vi "get_active_channels.vi"(7 "Trigger edge":bool[](array[boolean])=[FALSE, FALSE, FALSE, FALSE, FALSE, FALSE, FALSE, FALSE], 8 "Error In":errorcluster, 9 "swabian_local_data":T1={"events"={"update_status"=refnum, "update_chart"=refnum, "update_xy"=refnum, "send_channel_data"=refnum}, "stop_q"=refnum, "tagger_reference"=refnum, "connect_button"=refnum, "counter_reference"=refnum, "tagger_stream_reference"=refnum, "log_reference"=refnum, "current_log_offset"=0, "tt20_buffer_q"=refnum, "stream_to_file_button"=refnum, "num_records"=0, "connected?"=FALSE, "plots"=refnum, "histogram_bin_edges"=[], "histogrammer"=refnum, "plot_lifetimes"=refnum, "xy_graph"=refnum, "Reference\nChannel"=enum."ch0", "trigger_channels"=[], "filter_channels"=[], "active_channels"=[], "acq_mode"=0, "Reference\nChannel"=enum."ch0", "acq_time"=0, "sync_period_ps"=0, "raw_stream_path"=path "", "Leftovers"={"missing_sync_data"=[], "missing_events"=0}, "first_batch"=0, "first_sync_stamp"=0, "lifetime_settings"={"Plot Lifetimes"=FALSE, "start_time"=0.0, "stop_time"=0.0, "n_bins"=0, "Oscilloscope"=TRUE}, "Histogram_bins"=[], "last_processed_data"=[], "histogram_data"=[]}, 10 "Reference\nChannel":T3=enum."ch2", 11 "channels_to_stream":bool[](array[boolean])) -> (0 "Error In 2":errorcluster, 3 "swabian_local_data 2":T1={"events"={"update_status"=refnum, "update_chart"=refnum, "update_xy"=refnum, "send_channel_data"=refnum}, "stop_q"=refnum, "tagger_reference"=refnum, "connect_button"=refnum, "counter_reference"=refnum, "tagger_stream_reference"=refnum, "log_reference"=refnum, "current_log_offset"=0, "tt20_buffer_q"=refnum, "stream_to_file_button"=refnum, "num_records"=0, "connected?"=FALSE, "plots"=refnum, "histogram_bin_edges"=[], "histogrammer"=refnum, "plot_lifetimes"=refnum, "xy_graph"=refnum, "Reference\nChannel"=enum."ch0", "trigger_channels"=[], "filter_channels"=[], "active_channels"=[], "acq_mode"=0, "Reference\nChannel"=enum."ch0", "acq_time"=0, "sync_period_ps"=0, "raw_stream_path"=path "", "Leftovers"={"missing_sync_data"=[], "missing_events"=0}, "first_batch"=0, "first_sync_stamp"=0, "lifetime_settings"={"Plot Lifetimes"=FALSE, "start_time"=0.0, "stop_time"=0.0, "n_bins"=0, "Oscilloscope"=TRUE}, "Histogram_bins"=[], "last_processed_data"=[], "histogram_data"=[]})   [LabVIEW 2018]
uses:
  reference_checkbox_tdef.ctl
  swabian_local_data_tdef.ctl
  swabian_events_tdef.ctl
  update_chart_tdef.ctl
  channel_data_tdef.ctl
  C:/Users/SWIR TCSPC/Documents/swabian_LV/lib/TTCSharp32.dll
  lib/TTCSharp32.dll
  swabian_buffer_tdef.ctl
  lifetime_settings.ctl
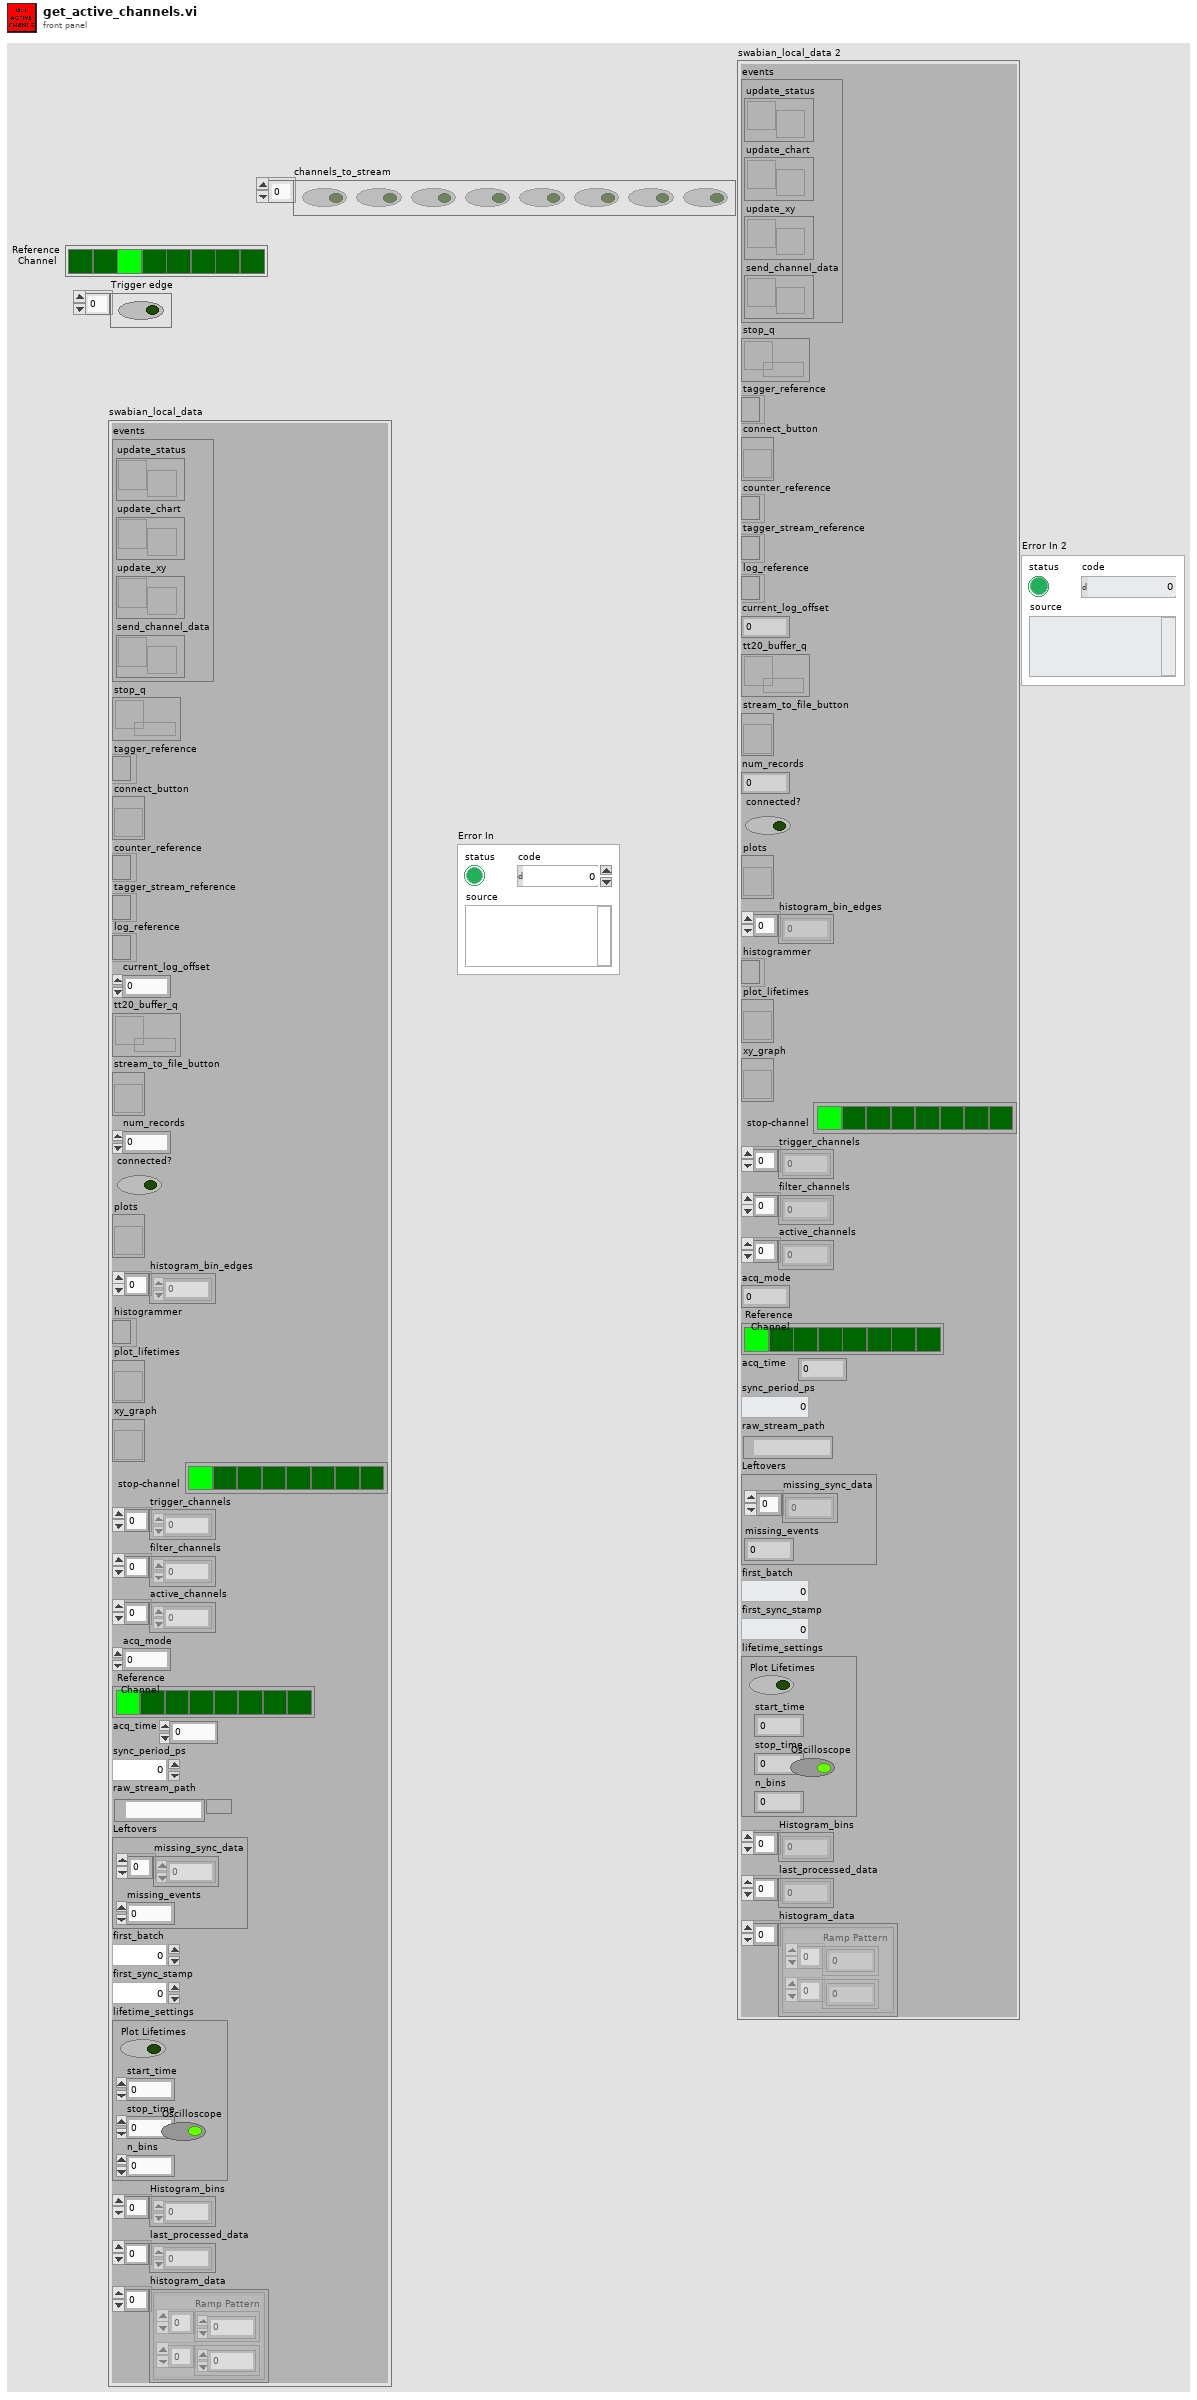
[diagram p1: front panel]
types:
  T1 = typedef "swabian_local_data_tdef.ctl" = cluster{"events":T2, "stop_q":refnum<queue>, "tagger_reference":refnum<k24>, "connect_button":refnum<vi>, "counter_reference":refnum<k24>, "tagger_stream_reference":refnum<k24>, "log_reference":refnum<file>, "current_log_offset":i64, "tt20_buffer_q":refnum<queue>, "stream_to_file_button":refnum<vi>, "num_records":u64, "connected?":bool, "plots":refnum<vi>, "histogram_bin_edges":i64[], "histogrammer":refnum<k24>, "plot_lifetimes":refnum<vi>, "xy_graph":refnum<vi>, "Reference\nChannel":T3, "trigger_channels":i32[], "filter_channels":i32[], "active_channels":i32[], "acq_mode":i32, "Reference\nChannel":T3, "acq_time":i64, "sync_period_ps":i64, "raw_stream_path":path, "Leftovers":cluster{"missing_sync_data":i64[], "missing_events":i32}, "first_batch":i32, "first_sync_stamp":i64, "lifetime_settings":T4, "Histogram_bins":dbl[], "last_processed_data":i64[], "histogram_data":cluster{"Ramp Pattern":dbl[], dbl[]}[]}
  T2 = typedef "swabian_events_tdef.ctl" = cluster{"update_status":refnum<user-event>, "update_chart":refnum<user-event>, "update_xy":refnum<user-event>, "send_channel_data":refnum<user-event>}
  T3 = typedef "reference_checkbox_tdef.ctl" = enum32{"No Selection", "ch0", "ch1", "ch2", "ch3", "ch4", "ch5", "ch6", "ch7"}
  T4 = typedef "lifetime_settings.ctl" = cluster{"Plot Lifetimes":bool, "start_time":dbl, "stop_time":dbl, "n_bins":i32, "Oscilloscope":bool}
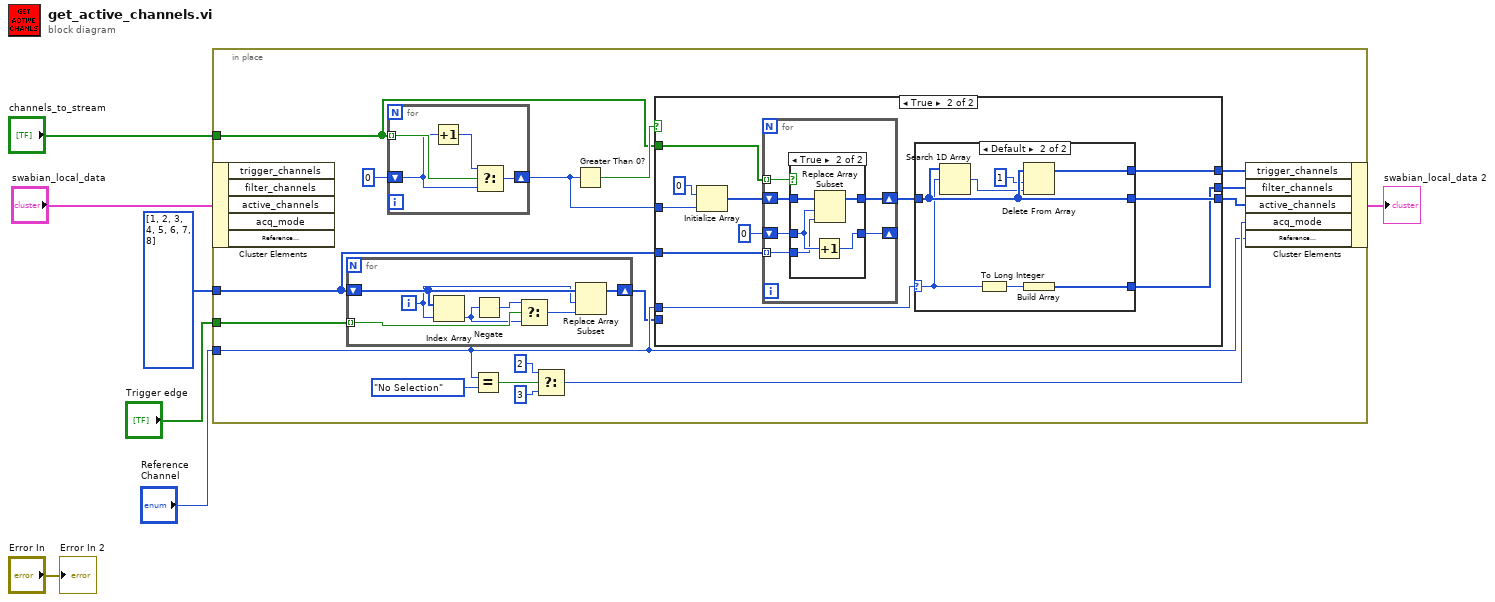
[diagram p0: block diagram]
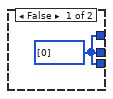
[diagram p2: hidden frame]
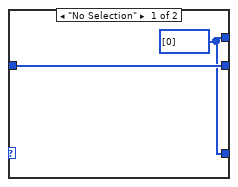
[diagram p4: hidden frame]
diagram:
  n1 = in-place {
    in-place-border: "channels_to_stream" -> [w10]
    in-place-border: "Reference\nChannel" -> [w16]
    in-place-border: i32[] [1, 2, 3, 4, 5, 6, 7, 8] -> [w9]
    in-place-border: "Trigger edge" -> [w15]
    n2 = in-place-cluster #1("swabian_local_data") -> ()  [unwired: 5 out]
    n3 = for {
      tunnel: w15 -> [w68] mode=indexing
      shift-right: [w62] -> w11
      shift-left: w9 -> [w66]
      i -> [w65]
      n4 = Index Array(array=w66, index=w65) -> (element=w64:i32)
      n5 = Negate(x=w64) -> (-x=w63:i32)
      n6 = Select(t=w63, s=w68, f=w64) -> (s? t:f=w67:i32)
      n7 = Replace Array Subset(array=w66, new element=w67, index=w65) -> (w62:i32[])
    }
    n8 = for {
      tunnel: w10 -> [w61] mode=indexing
      shift-right: [w59] -> w12
      shift-left: 0 -> [w58]
      n9 = Increment(x=w58) -> (x+1=w60:i32)
      n10 = Select(t=w60, s=w61, f=w58) -> (s? t:f=w59:i32)
    }
    n11 = Equal?(x=w16, y=reference_checkbox_tdef."No Selection") -> (x = y?=w22:bool)
    n12 = Select(t=2, s=w22, f=3 ("t")) -> (s? t:f=w19:i32)
    n13 = Greater Than 0?(x=w12) -> (x > 0?=w13:bool)
    n14 = case shown="True" w13 {
      tunnel: [w24 w35] -> w8
      tunnel: [w24 w34] -> w18
      tunnel: [w24 w33] -> w17
      tunnel: w16 -> [_ w32]
      tunnel: w12 -> [_ w31]
      tunnel: w11 -> [_ _]
      tunnel: w10 -> [_ w29]
      tunnel: w9 -> [_ w28]
      frame False {
        w24 = i32[] [0]
      }
      frame True {
        n15 = Initialize Array(0 ("element"), w31) -> (w27:i32[])
        n16 = for {
          tunnel: w29 -> [w41] mode=indexing
          tunnel: w28 -> [w39] mode=indexing
          shift-right: [w38] -> w25
          shift-left: w27 -> [w40]
          shift-right: [w36] -> _
          shift-left: 0 -> [w37]
          n17 = case shown="True" w41 {
            tunnel: w40 -> [w43 w48]
            tunnel: w39 -> [_ w44]
            tunnel: [w43 w47] -> w38
            tunnel: w37 -> [w42 w45]
            tunnel: [w42 w46] -> w36
            frame False {
            }
            frame True {
              n18 = Increment(x=w45) -> (x+1=w46:i32)
              n19 = Replace Array Subset(array=w48, new element=w44, index=w45) -> (w47:i32[])
            }
          }
        }
        n20 = case shown="Default" w32 {
          selector: w32 -> [_ w51]
          tunnel: w25 -> [w50 w57]
          tunnel: [w50 w57] -> w35
          tunnel: [w49 w54] -> w34
          tunnel: [w49 w53] -> w33
          frame "No Selection" {
            w49 = i32[] [0]
          }
          frame Default {
            n21 = Search 1D Array(1D array=w57, element=w51) -> (index of element=w55:i32)  [unwired: 1 in]
            n22 = To Long Integer(number=w51) -> (32bit integer=w52:i32)
            n23 = Delete From Array(array=w57, length=1, index=w55) -> (array with subset deleted=w54:i32[])  [unwired: 1 out]
            n24 = Build Array(w52) -> (w53:i32[])
          }
        }
      }
    }
    n25 = in-place-cluster #1("trigger_channels"=w18, "filter_channels"=w17, "active_channels"=w8, "acq_mode"=w19, "Reference\nChannel"=w16) -> (→"swabian_local_data 2":T1)
  }
  "Error In 2" <- "Error In"
